vi "Watlow Read.vi"(0 "Adress":u8=3 format="%x", 1 "Register":u32, 3 "error in":errorcluster, 4 "VISA resource name":refnum<visa-resource-name>="ASRL2::INSTR") -> (5 "Number":u32, 6 "error out":errorcluster)   [LabVIEW 2009]
uses:
  <vilib>/Instr/_visa.llb/VISA Configure Serial Port (Instr).vi
panel:
  out "Serial Settings:Number of Bytes at Serial Port":u32
  out "write buffer 2":string
  out "unsigned byte array":u8[](array[numeric]) format="%x"
  out "Reg L":u8=100
  out "Reg H":u8
  out "Read buffer":string
  # "064h- Temper\n12Ch- Set Point"
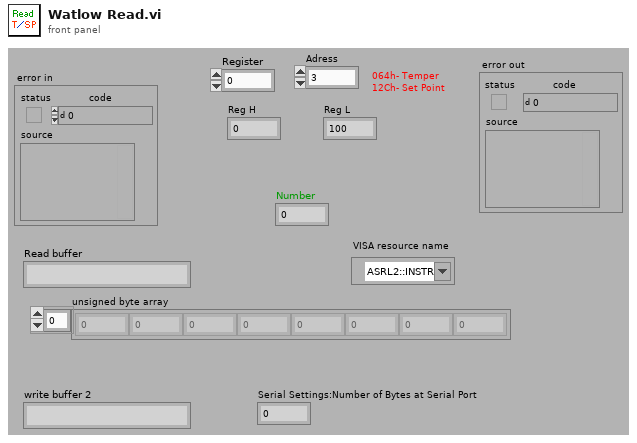
[diagram p1: front panel]
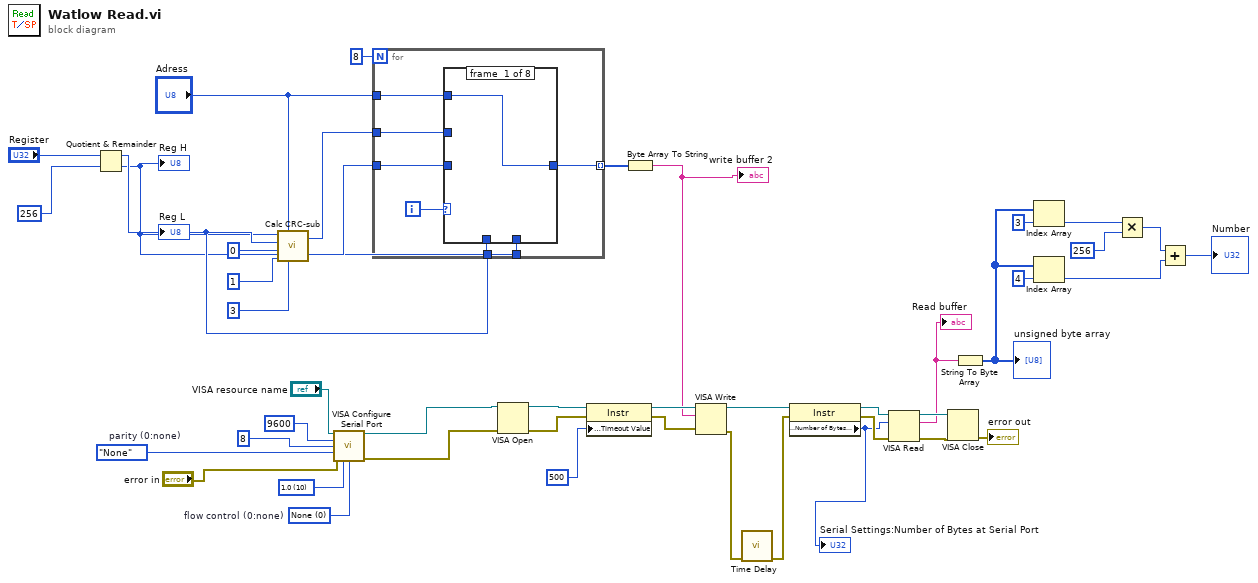
[diagram p0: block diagram]
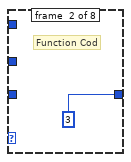
[diagram p2: hidden frame]
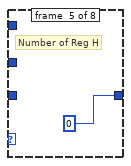
[diagram p5: hidden frame]
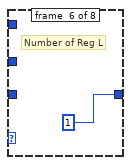
[diagram p6: hidden frame]
diagram:
  w10 = enum16{"None", "Odd", "Even", "Mark", "Space"}."None"  # parity (0:none)
  w6 = u16 0 items=["None"=0, "XON/XOFF"=1, "RTS/CTS"=2, "DTR/DSR"=4]  # flow control (0:none)
  w7 = u16 10 items=["1.0"=10, "1.5"=15, "2.0"=20] ("stop bits (10: 1 bit)")
  n1 = Quotient & Remainder(x="Register", y=u32 256) -> (x-y*floor(x/y)=w12:u32, floor(x/y)=w11:u32)
  "Reg H" <- w11
  "Reg L" <- w12
  n2 = call "Calc CRC-sub.vi"("Command"=u8 3, "Adress"="Adress", "Data L"=u8 1 ("NR-L"), "Data H"=u8 0 ("NR-H"), "Reg L"=w12, "Reg H"=w11) -> ("L byte"=w30:u8, "H byte"=w29:u8)
  n3 = call-poly "VISA Configure Serial Port"("VISA resource name"="VISA resource name", "baud rate (9600)"=u32 9600, "data bits (8)"=u16 8, "parity (0:none)"=w10, "error in (no error)"="error in", "stop bits (10: 1 bit)"=w7, "flow control (0:none)"=w6) -> ("VISA resource name out"=w3:refnum<visa-resource-name>, "error out"=w2:errorcluster)  [unwired: 7 out]
  n4 = for {
    N: 8 -> [_]
    tunnel: [w51] -> w45 mode=indexing
    tunnel: "Adress" -> [w50]
    tunnel: w30 -> [w49]
    tunnel: w29 -> [w48]
    tunnel: w12 -> [w47]
    tunnel: w11 -> [w46]
    i -> [w52]
    n5 = case shown="0, Default" w52 {
      tunnel: [w53 u8 3 ("Command") w55 w56 u8 0 ("NR-H") u8 1 ("NR-L") w59 w60] -> w51
      tunnel: w50 -> [w53 _ _ _ _ _ _ _]
      tunnel: w49 -> [_ _ _ _ _ _ w59 _]
      tunnel: w48 -> [_ _ _ _ _ _ _ w60]
      tunnel: w47 -> [_ _ _ w56 _ _ _ _]
      tunnel: w46 -> [_ _ w55 _ _ _ _ _]
      frame #0 {
      }
      frame #1 {
        # "Function Cod"
      }
      frame #2 {
        # "Start Reg H"
      }
      frame #3 {
        # "Start Reg L"
      }
      frame #4 {
        # "Number of Reg H"
      }
      frame #5 {
        # "Number of Reg L"
      }
      frame #6 {
        # "CRC - L"
      }
      frame #7 {
        # "CRC- H"
      }
    }
  }
  n6 = VISA Open(error in (no error)=w2, VISA resource name=w3) -> (VISA resource name=w41:refnum<visa-resource-name>, error out=w40:errorcluster)  [unwired: 3 out]
  n7 = property class="Instr"(reference=w41, error in=w40, "General Settings:Timeout Value"=u32 500) -> (reference out=w39:refnum<visa-resource-name>, error out=w38:errorcluster)
  n8 = Byte Array To String(unsigned byte array=w45) -> (string=w20:string)
  "write buffer 2" <- w20
  n9 = VISA Write(VISA resource name=w39, write buffer=w20, error in (no error)=w38) -> (VISA resource name out=w17:refnum<visa-resource-name>, error out=w19:errorcluster)  [unwired: 1 out]
  n10 = call "Time Delay"("error in (no error)"=w19) -> ("error out"=w18:errorcluster)  [unwired: 1 in, 9 out]
  n11 = property on="Property Node" class="Instr"(reference=w17, error in=w18) -> (reference out=w16:refnum<visa-resource-name>, error out=w15:errorcluster, "Serial Settings:Number of Bytes at Serial Port"=w1:u32)
  "Serial Settings:Number of Bytes at Serial Port" <- w1
  n12 = VISA Read(VISA resource name=w16, byte count=w1, error in (no error)=w15) -> (VISA resource name out=w37:refnum<visa-resource-name>, read buffer=w35:string, error out=w36:errorcluster)  [unwired: 1 out]
  "Read buffer" <- w35
  n13 = VISA Close(VISA resource name=w37, error in (no error)=w36) -> (error out=→"error out":errorcluster)
  n14 = String To Byte Array(string=w35) -> (unsigned byte array=w28:u8[])
  "unsigned byte array" <- w28
  n15 = Index Array(array=w28, index=3) -> (element=w25:u8)
  n16 = Index Array(array=w28, index=4) -> (element=w22:u8)
  n17 = Multiply(x=w25, y=u32 256) -> (x*y=w23:u32)
  n18 = Add(x=w23, y=w22) -> (x+y=→"Number":u32)
